vi "Controller Close Synchronization Objects.vi"(8 "error in (no error)":errorcluster, 11 "Sync Objects":T3) -> (0 "error out":errorcluster)   [LabVIEW 2011, in "Controller VIs.lvlib"]
uses:
  Controller VIs.lvlib
  Types Definitions/Type Synchronization Objects.ctl
  Types Definitions/Type Blocking Synchronization Objects.ctl
  Types Definitions/Type Monitoring Data.ctl
  Types Definitions/Type Operation Mode State.ctl
  Types Definitions/Type Diagnostics Data.ctl
  Types Definitions/Type CPU Loads Array.ctl
  Types Definitions/Type CPU Loads.ctl
  Types Definitions/Type Non-blocking Synchronization Objects.ctl
  Types Definitions/Type FOFB Variables.ctl
  Types Definitions/Type Actuation State.ctl
  Misc VIs.lvlib
  Type Definitions.lvlib
panel:
  out "Non-blocking":T1
  out "Blocking":T2
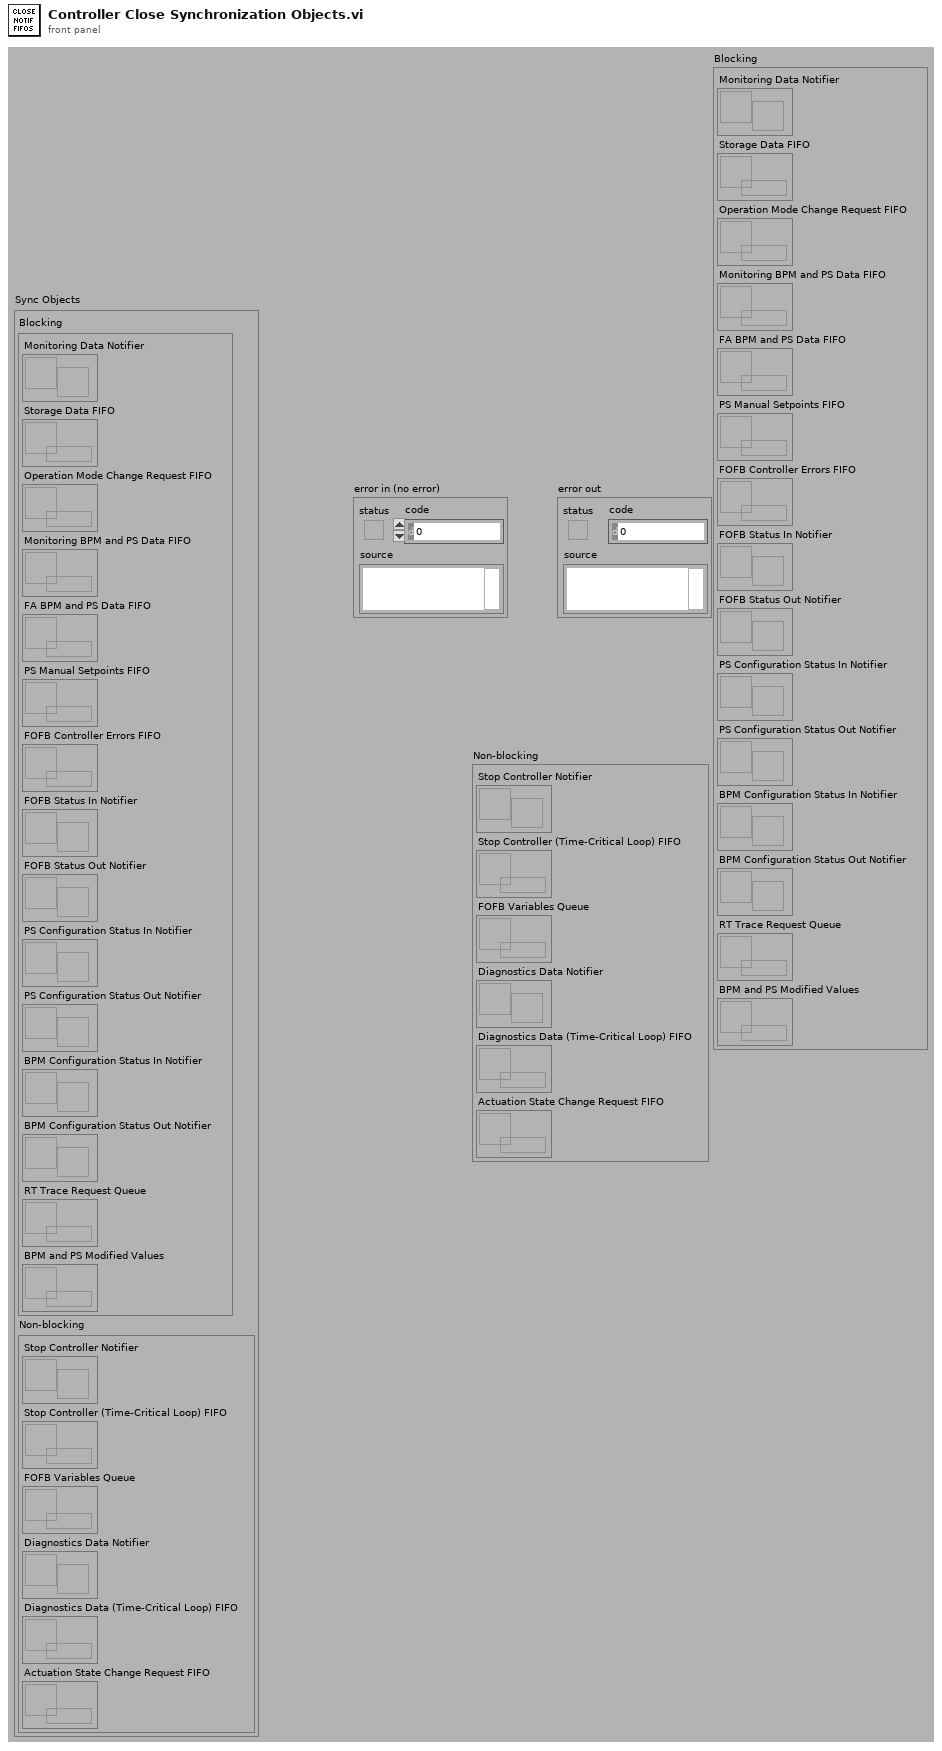
[diagram p1: front panel]
types:
  T1 = typedef "Type Definitions.lvlib/Type Non-blocking Synchronization Objects.ctl" = cluster{"Stop Controller Notifier":refnum<notifier>, "Stop Controller (Time-Critical Loop) FIFO":refnum<k33>, "FOFB Variables Queue":refnum<queue>, "Diagnostics Data Notifier":refnum<notifier>, "Diagnostics Data (Time-Critical Loop) FIFO":refnum<k33>, "Actuation State Change Request FIFO":refnum<k33>}
  T2 = typedef "Type Definitions.lvlib/Type Blocking Synchronization Objects.ctl" = cluster{"Monitoring Data Notifier":refnum<notifier>, "Storage Data FIFO":refnum<queue>, "Operation Mode Change Request FIFO":refnum<k33>, "Monitoring BPM and PS Data FIFO":refnum<k33>, "FA BPM and PS Data FIFO":refnum<k33>, "PS Manual Setpoints FIFO":refnum<k33>, "FOFB Controller Errors FIFO ":refnum<k33>, "FOFB Status In Notifier":refnum<notifier>, "FOFB Status Out Notifier":refnum<notifier>, "PS Configuration Status In Notifier":refnum<notifier>, "PS Configuration Status Out Notifier":refnum<notifier>, "BPM Configuration Status In Notifier":refnum<notifier>, "BPM Configuration Status Out Notifier":refnum<notifier>, "RT Trace Request Queue":refnum<queue>, "BPM and PS Modified Values":refnum<k33>}
  T3 = typedef "Type Definitions.lvlib/Type Synchronization Objects.ctl" = cluster{"Blocking":T2, "Non-blocking":T1}
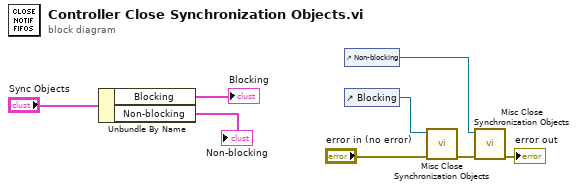
[diagram p0: block diagram]
diagram:
  n1 = Unbundle By Name("Sync Objects") -> ("Blocking"=→"Blocking":T2, "Non-blocking"=→"Non-blocking":T1)
  n2 = control-ref of="Non-blocking"() -> (w1:refnum<vi>)
  n3 = control-ref of="Blocking"() -> (w2:refnum<vi>)
  n4 = call "Misc Close Synchronization Objects.vi"("error in (no error)"="error in (no error)", "Cluster Reference"=w2) -> ("error out"=w5:errorcluster)  [unwired: 9 in]
  n5 = call "Misc Close Synchronization Objects.vi"("error in (no error)"=w5, "Cluster Reference"=w1) -> ("error out"=→"error out":errorcluster)  [unwired: 9 in]
